vi "SNMP Get Request.vi"(6 "UDP Port":u16=161, 7 "IP Address":string="128.193.66.74", 8 "error in (no error)":errorcluster, 9 "OID ARRAY":string[](array[string]), 10 "Community Name":string="public", 11 "connection ID":refnum<k16>) -> (0 "error out":errorcluster, 2 "RequestID":u16 format="%.0x", 3 "connection ID":refnum<k16>)   [LabVIEW 2017]
doc: "This VI builds a SNMP Get PDU and sends it to the specified agent. The VI accepts an array of OIDs which will specify the data to retrieve."
panel:
  out "Outgoing SNMP PAcket":u8[](array[numeric]) format="%.0x"
  out "Snmp Packet length":i32
  out "net address":u32
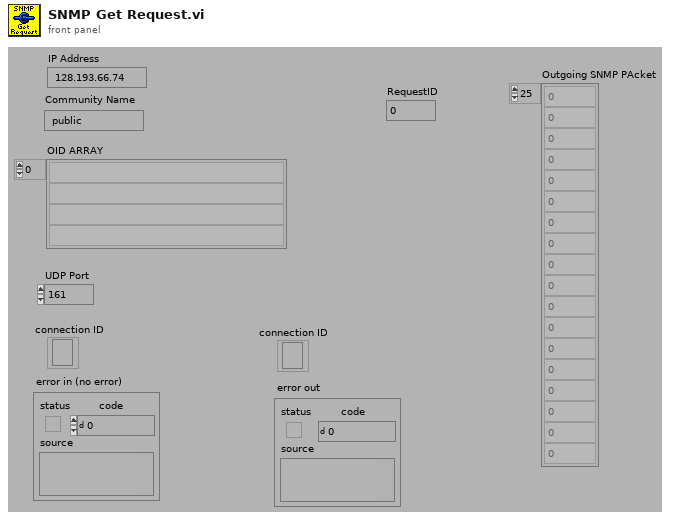
[diagram p1: front panel]
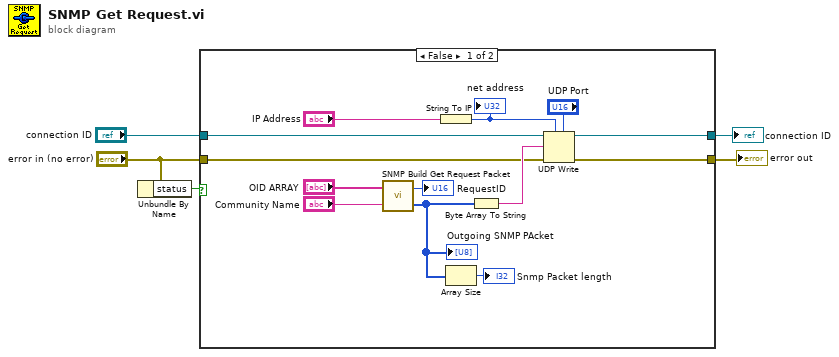
[diagram p0: block diagram]
diagram:
  n1 = Unbundle By Name("error in (no error)") -> ("status"=w3:bool)
  n2 = case shown="False" w3 {
    tunnel: [w13 w20] -> w5
    tunnel: "connection ID" -> [w10 w20]
    tunnel: "error in (no error)" -> [w9 w19]
    tunnel: [w8 w19] -> w1
    frame False {
      n3 = call "SNMP Build Get Request Packet.vi"("Community Name"="Community Name", "OID ARRAY"="OID ARRAY") -> ("SNMP Packet"=w15:u8[], "RequestID"=→"RequestID":u16)
      "Outgoing SNMP PAcket" <- w15
      n4 = String To IP(1:"IP Address") -> (0:w11:u32)
      "net address" <- w11
      n5 = Array Size(array=w15) -> (size(s)=→"Snmp Packet length":i32)
      n6 = Byte Array To String(unsigned byte array=w15) -> (string=w18:string)
      n7 = UDP Write(address=w11, port or service name="UDP Port", connection ID=w10, data in=w18, 8:w9) -> (error out=w8:errorcluster, 3:w13:refnum<k16>)  [unwired: 1 out]
    }
    frame True {
    }
  }
  "connection ID" <- w5
  "error out" <- w1
